vi "set_repetitions.vi"(8 "error in (no error)":errorcluster, 10 "repetitions":i32, 11 "GenericTrajectory in":refnum<class "GenericTrajectory.lvclass">) -> (0 "error out":errorcluster, 3 "GenericTrajectory out":refnum<class "GenericTrajectory.lvclass">)   [LabVIEW 2010, in "GenericTrajectory.lvclass"]
doc: "sets the number of times the cycle has to be scanned repeatedly when in single-sweep mode or experiment mode"
uses:
  GenericTrajectory.lvclass
  GenericTrajectory.lvclass/GenericTrajectory.ctl
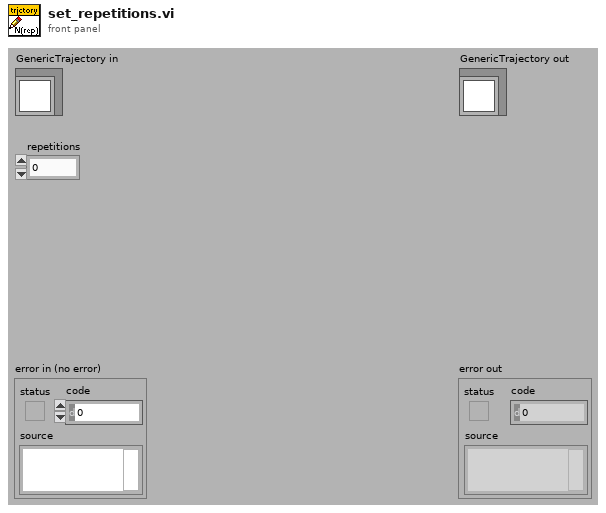
[diagram p1: front panel]
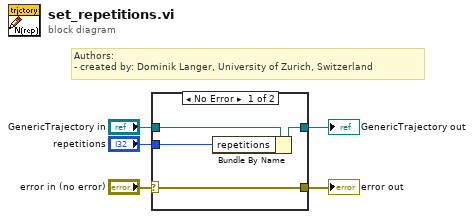
[diagram p0: block diagram]
diagram:
  # "Authors: \n- created by: Dominik Langer, University of Zurich, Switzerland"
  n1 = case shown="No Error" "error in (no error)" {
    selector: "error in (no error)" -> [w9 w10]
    tunnel: [w9 w10] -> w4
    tunnel: [w7 w11] -> w2
    tunnel: "GenericTrajectory in" -> [w8 w11]
    tunnel: "repetitions" -> [w6 _]
    frame No Error {
      n2 = Bundle By Name(cluster=w8, "repetitions"=w6) -> (w7:refnum<class "GenericTrajectory.lvclass">)
    }
    frame Error {
    }
  }
  "error out" <- w4
  "GenericTrajectory out" <- w2
